vi "LVClass_WavefrontCorrector CheckRelativePositionSaturation.vi"(0 "WavefrontCorrector in":refnum<class "WavefrontCorrector.lvclass">, 5 "Relative Positions":T1, 11 "error in (no error)":errorcluster) -> (4 "WavefrontCorrector out":refnum<class "WavefrontCorrector.lvclass">, 6 "Relative Positions OUT":T1, 8 "saturated_act_count":i32, 15 "error out":errorcluster)   [LabVIEW 2020, in "WavefrontCorrector.lvclass"]
doc: "Assert if requested relative positions satisfy current preferences.\n\n--------------------------------------------------------------------------------\n\n<B>correctorIn </B> : WavefrontCorrector object.\n<B>correctorOut </B> : WavefrontCorrector object.\n<B>position </B> : Requested relatives positions.\n<B>ErrorIn </B> : Error\n<B>ErrorOut </B> : Error\n\n--------------------------------------------------------------------------------"
uses:
  WavefrontCorrector.lvclass
  Controls/Wavefront Corrector Position.ctl
  WavefrontCorrector.lvclass/WavefrontCorrector.ctl
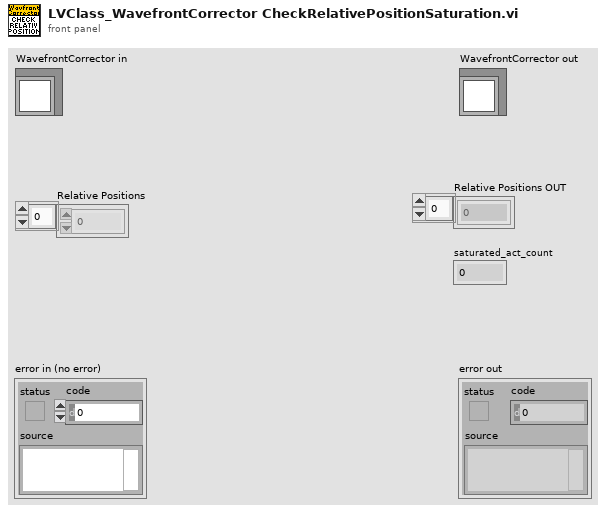
[diagram p1: front panel]
types:
  T1 = typedef "Wavefront Corrector Position.ctl" = sgl[]
  T2 = typedef "ClassID.ctl" = i64
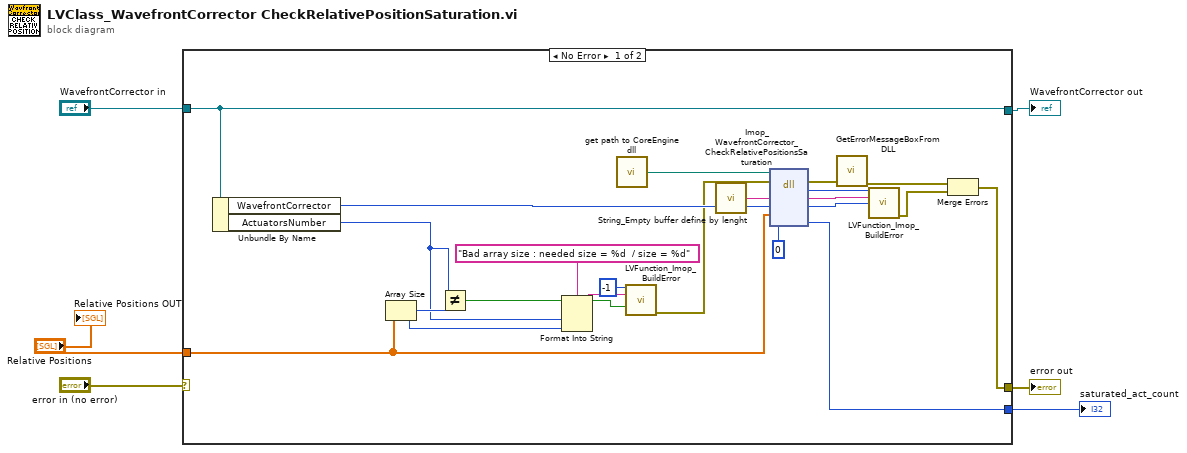
[diagram p0: block diagram]
diagram:
  n1 = case shown="No Error" "error in (no error)" {
    selector: "error in (no error)" -> [_ w29]
    tunnel: [w19 w29] -> w3
    tunnel: [w18 w28] -> w4
    tunnel: "WavefrontCorrector in" -> [w18 w28]
    tunnel: "Relative Positions" -> [w10 _]
    tunnel: [w9 _] -> w1
    frame No Error {
      n2 = Unbundle By Name(w18) -> ("WavefrontCorrector"=w20:T2, "ActuatorsNumber"=w12:i32)
      n3 = Array Size(array=w10) -> (size(s)=w15:i32)
      n4 = Not Equal?(x=w12, y=w15) -> (x != y?=w14:bool)
      n5 = Format Into String(format string="Bad array size : needed size = %d  / size = %d" ("String to Prepend to source (\"\")"), w12, w15) -> (resulting string=w16:string)  [unwired: 2 in, 1 out]
      n6 = call "get path to CoreEngine dll.vi"() -> ("path to wavekit library"=w24:path)  [unwired: 14 in, 1 out]
      n7 = call "LVFunction_Imop_BuildError.vi"("code"=-1, "String to Prepend to source (\"\")"=w16, "Activate error? (true)"=w14) -> ("error out"=w11:errorcluster)  [unwired: 12 in]
      n8 = call "String_Empty buffer define by lenght.vi"() -> ("Empty buffer"=w25:string)  [unwired: 1 in]
      n9 = dll-call lib="D:/soft/HASO_v3/SVN_trunk/ImOpCoreEngine4_LV2011/DLLs/c_interface_vc100.dll" fn="Imop_WavefrontCorrector_CheckRelativePositionsSaturation"(path in=w24, error in=w11, "message"=w25, "WavefrontCorrection"=w20, "Relative Position"=w10, "saturated_act_count"=0) -> (error out=w23:errorcluster, "return type"=w27:i32, "message"=w26:string, "WavefrontCorrection"=w7:i64, "saturated_act_count"=w9:i32)  [unwired: 2 in, 1 out]
      n10 = call "GetErrorMessageBoxFromDLL.vi"("error IN"=w23) -> ("error OUT"=w22:errorcluster)  [unwired: 10 in]
      n11 = call "LVFunction_Imop_BuildError.vi"("code"=w27, "String to Prepend to source (\"\")"=w26, "Adresse"=w7) -> ("error out"=w21:errorcluster)  [unwired: 12 in]
      n12 = Merge Errors(w22, w21) -> (w19:errorcluster)
    }
    frame Error {
    }
  }
  "error out" <- w3
  "WavefrontCorrector out" <- w4
  "saturated_act_count" <- w1
  "Relative Positions OUT" <- "Relative Positions"
